vi "Set Default LabVIEW Printer.vi"(10 "Model Number":string="p700") -> (1 "Array of Missing Printer":string[](array[string]), 2 "Found?":bool)   [LabVIEW 2016]
uses:
  FP DAQ/UTILS/Array String Contains.vi
panel:
  out "Printing:Default Printer 2":string
  out "Printing:Default Printer":string
  out "Matched String":string
  out "Array - String":string[](array[string])
  in  "Error In":errorcluster
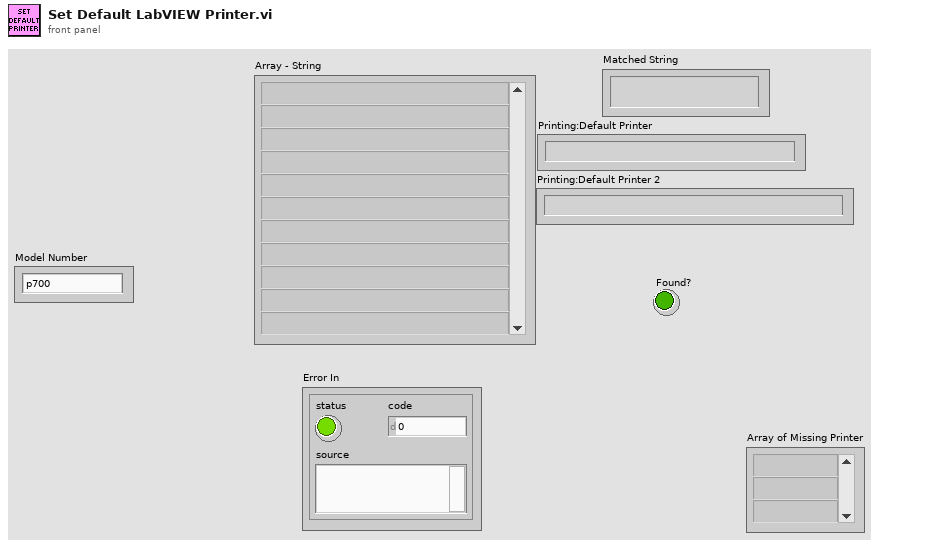
[diagram p1: front panel]
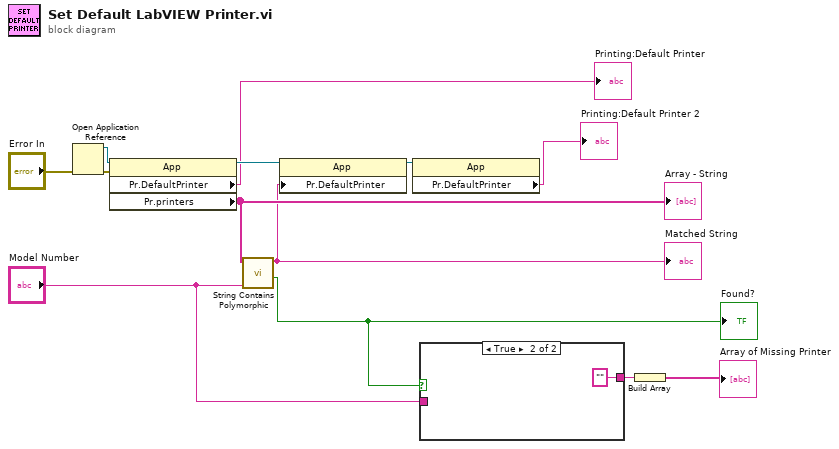
[diagram p0: block diagram]
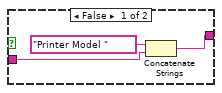
[diagram p2: hidden frame]
diagram:
  n1 = Open Application Reference(8:"Error In") -> (0:w11:errorcluster, 3:w12:refnum<vi>)  [unwired: 3 in]
  n2 = property class="App"(reference=w12, error in=w11) -> (reference out=w10:refnum<vi>, "Pr.DefaultPrinter"=→"Printing:Default Printer":string, "Pr.printers"=w9:string[])  [unwired: 1 out]
  "Array - String" <- w9
  n3 = call-poly "String Contains Polymorphic.vi"("Regular expression"="Model Number", "Array - String"=w9) -> ("Found?"=w1:bool, "Matched String"=w8:string)  [unwired: 4 in]
  "Matched String" <- w8
  "Found?" <- w1
  n4 = property class="App"(reference=w10, "Pr.DefaultPrinter"=w8) -> (reference out=w6:refnum<vi>)  [unwired: 1 in, 1 out]
  n5 = property class="App"(reference=w6) -> ("Pr.DefaultPrinter"=→"Printing:Default Printer 2":string)  [unwired: 1 in, 2 out]
  n6 = case shown="True" w1 {
    tunnel: "Model Number" -> [w15 _]
    tunnel: [w14 ""] -> w3
    frame False {
      n7 = Concatenate Strings("Printer Model " ("string"), w15) -> (w14:string)
    }
    frame True {
    }
  }
  n8 = Build Array(w3) -> (→"Array of Missing Printer":string[])
